vi "SetComparison.vi"(8 "error in":errorcluster, 10 "Comparison":string, 11 "StringMeasureLimit in":refnum<class "StringMeasureLimit.lvclass">) -> (0 "error out":errorcluster, 3 "StringMeasureLimit out":refnum<class "StringMeasureLimit.lvclass">)   [LabVIEW 2021, in "ProligentXMLGenerator.lvlib" / "StringMeasureLimit.lvclass"]
doc: "Real Measure Limit Comparison Type"
uses:
  StringMeasureLimit.lvclass
  StringMeasureLimit.lvclass/StringMeasureLimit.ctl
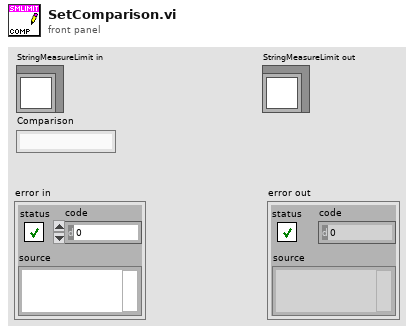
[diagram p1: front panel]
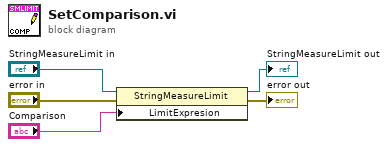
[diagram p0: block diagram]
diagram:
  n1 = property class="StringMeasureLimit"(reference="StringMeasureLimit in", error in="error in", "LimitExpresion"="Comparison") -> (reference out=→"StringMeasureLimit out":refnum<class "StringMeasureLimit.lvclass">, error out=→"error out":errorcluster)
